vi "VI Tree.vi"   [LabVIEW 2012, in "Phidget PH Sensor.lvlib"]
doc: "${PHSensor:VITreeHeader}"
uses:
  <instrlib>/Phidgets/Phidget PH Sensor/Phidget PH Sensor.lvlib
  <instrlib>/Phidgets/Phidget PH Sensor/Public/PHSensorStart.vi
  <instrlib>/Phidgets/Phidget PH Sensor/Public/PHSensorOpen.vi
  <instrlib>/Phidgets/Phidget PH Sensor/Public/PHSensorClose.vi
panel:
  # "(c) 2015 Phidgets Inc..  ALL RIGHTS RESERVED."
  # "SEE DIAGRAM\nFOR VI TREE."
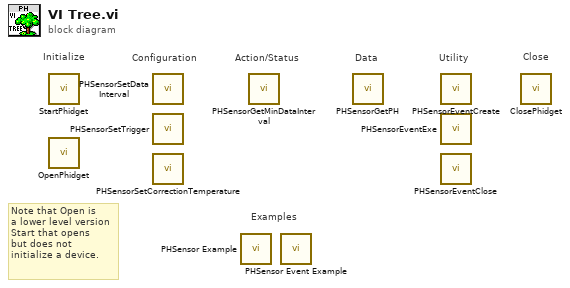
[diagram p0: block diagram]
diagram:
  # "Note that Open is\na lower level version\nStart that opens\nbut does not \ninitialize a device."
  # "Examples"
  # "Configuration"
  # "Utility"
  # "Data"
  # "Action/Status"
  # "Close"
  # "Initialize"
  n1 = call-poly <instrlib>:"StartPhidget.vi"() -> ()  [unwired: 12 in, 4 out]
  n2 = call-poly <instrlib>:"OpenPhidget.vi"() -> ()  [unwired: 8 in, 4 out]
  n3 = call <instrlib>:"PHSensorSetDataInterval.vi"() -> ()  [unwired: 9 in, 2 out]
  n4 = call <instrlib>:"PHSensorSetTrigger.vi"() -> ()  [unwired: 9 in, 2 out]
  n5 = call <instrlib>:"PHSensorSetCorrectionTemperature.vi"() -> ()  [unwired: 9 in, 2 out]
  n6 = call <instrlib>:"PHSensor Example.vi"() -> ()  [unwired: 12 in]
  n7 = call <instrlib>:"PHSensorGetMinDataInterval.vi"() -> ()  [unwired: 8 in, 3 out]
  n8 = call <instrlib>:"PHSensor Event Example.vi"() -> ()  [unwired: 12 in]
  n9 = call <instrlib>:"PHSensorGetPH.vi"() -> ()  [unwired: 8 in, 3 out]
  n10 = call <instrlib>:"PHSensorEventCreate.vi"() -> ()  [unwired: 9 in, 3 out]
  n11 = call <instrlib>:"PHSensorEventExe.vi"() -> ()  [unwired: 5 in, 7 out]
  n12 = call <instrlib>:"PHSensorEventClose.vi"() -> ()  [unwired: 10 in, 2 out]
  n13 = call-poly <instrlib>:"ClosePhidget.vi"() -> ()  [unwired: 11 in, 1 out]
